vi "Mechanical Action of a Boolean Control.vi"() -> ()   [LabVIEW 2022 SP3]
panel:
  in  "Boolean":bool
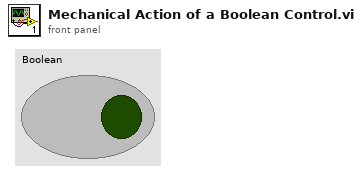
[diagram p1: front panel]
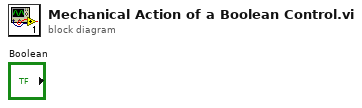
[diagram p0: block diagram]
diagram:
